vi "LS330_ReadFile.vi"(8 "error in":errorcluster, 9 "File Exists?":bool, 11 "refnum":refnum<file>) -> (0 "error out":errorcluster, 1 "Cluster":T1, 3 "refnum out":refnum<file>)   [LabVIEW 2021]
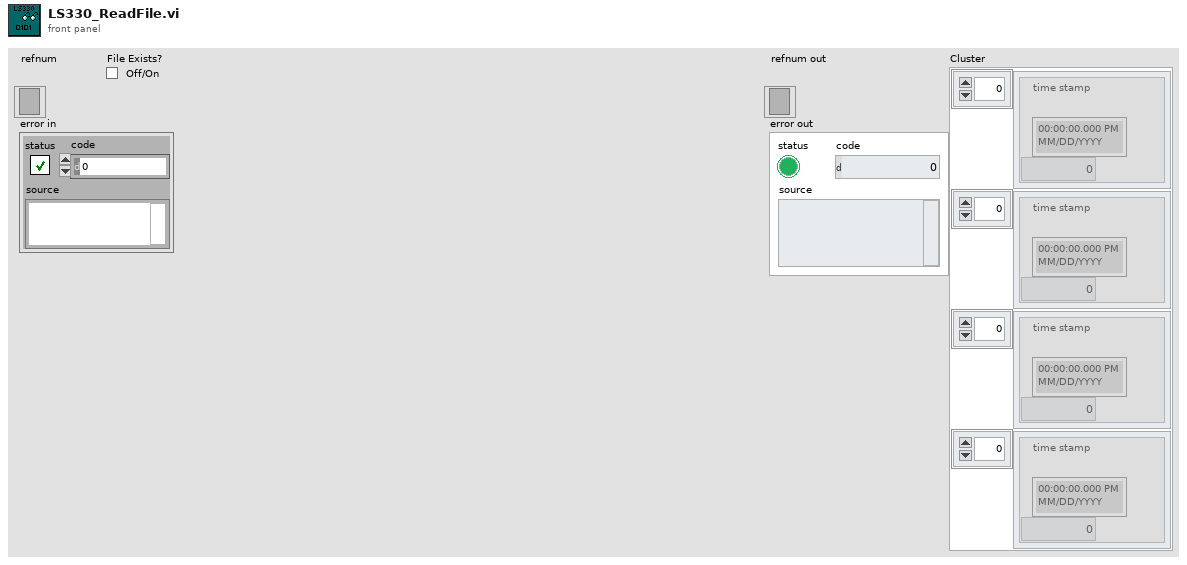
[diagram p1: front panel]
types:
  T1 = cluster{"Array":cluster{"time stamp":timestamp, "Numeric":dbl}[], "Array":cluster{"time stamp":timestamp, "Numeric":dbl}[], "Array":cluster{"time stamp":timestamp, "Numeric":dbl}[], "Array":cluster{"time stamp":timestamp, "Numeric":dbl}[]}
  T2 = cluster{cluster{"time stamp":timestamp, dbl}[], cluster{"time stamp":timestamp, dbl}[], cluster{"time stamp":timestamp, dbl}[], cluster{"time stamp":timestamp, dbl}[]}
  T3 = typedef "LVDateTimeRec.ctl" = cluster{"fractional second":dbl, "second":i32, "minute":i32, "hour":i32, "day of month":i32, "month":i32, "year":i32, "day of week":i32, "day of year":i32, "DST":i32}
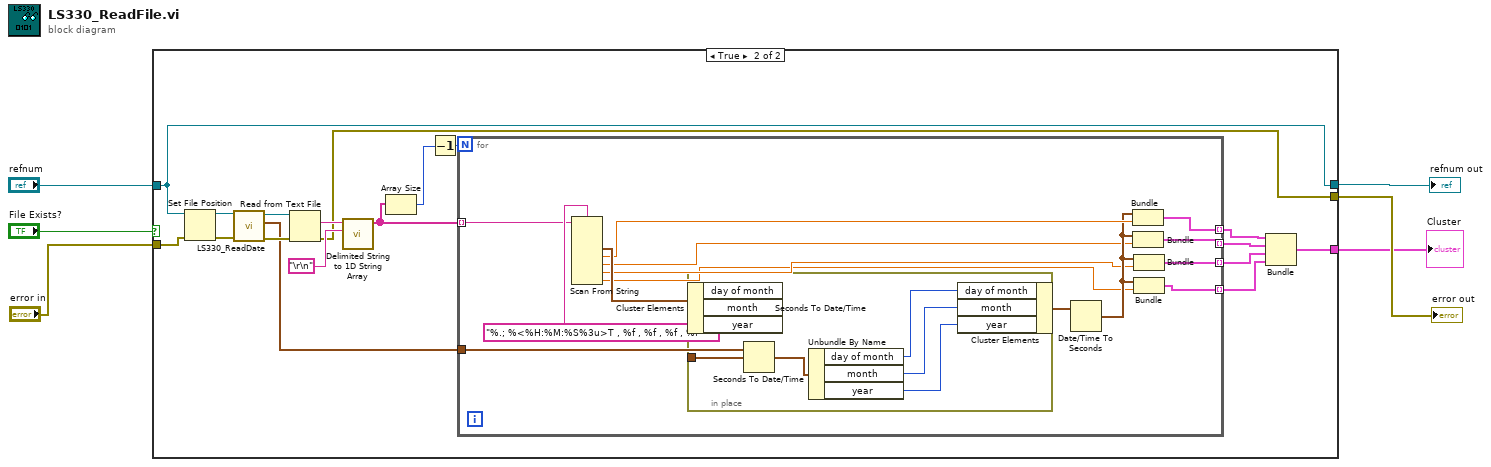
[diagram p0: block diagram]
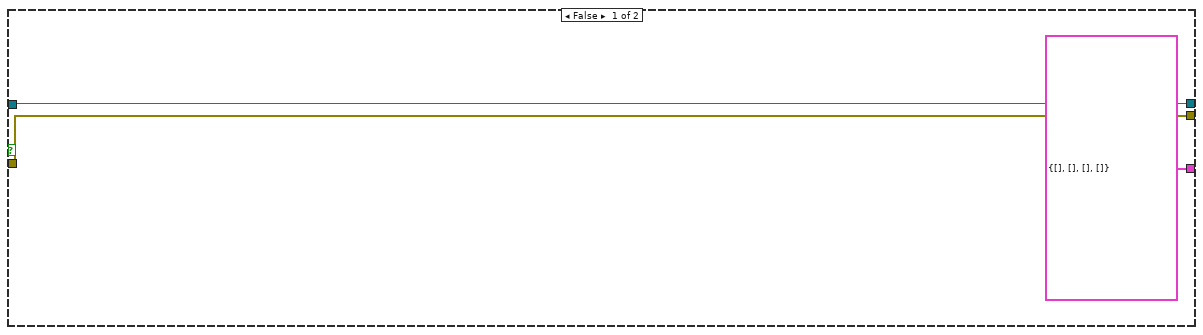
[diagram p2: hidden frame]
diagram:
  n1 = case shown="True" "File Exists?" {
    tunnel: "error in" -> [w8 w27]
    tunnel: "refnum" -> [w9 w15]
    tunnel: [w9 w15] -> w5
    tunnel: [w8 w16] -> w4
    tunnel: [T2 {[], [], [], []} w10] -> w1
    frame False {
    }
    frame True {
      n2 = Set File Position(refnum=w15, error in=w27) -> (refnum out=w26:refnum<file>, error out=w25:errorcluster)  [unwired: 2 in]
      n3 = call "LS330_ReadDate.vi"("error in"=w25, "refnum"=w26) -> ("error out"=w23:errorcluster, "Date"=w22:timestamp, "refnum 2"=w24:refnum<file>)  [unwired: 7 in]
      n4 = Read from Text File(file (use dialog)=w24, error in=w23) -> (text=w21:string, error out=w16:errorcluster)  [unwired: 2 in, 2 out]
      n5 = call <vilib>:"Delimited String to 1D String Array.vi"("delimiter"="\r\n", "delimited string"=w21) -> ("string array"=w19:string[])  [unwired: 9 in]
      n6 = Array Size(array=w19) -> (size(s)=w17:i32)
      n7 = Decrement(x=w17) -> (x-1=w18:i32)
      n8 = for {
        N: w18 -> [_]
        tunnel: w22 -> [w43]
        tunnel: w19 -> [w38] mode=indexing
        tunnel: [w36] -> w14 mode=indexing
        tunnel: [w30] -> w13 mode=indexing
        tunnel: [w29] -> w12 mode=indexing
        tunnel: [w28] -> w11 mode=indexing
        n9 = Scan From String(format string="%.; %<%H:%M:%S%3u>T , %f , %f , %f , %f", input string=w38) -> (output 1=w41:timestamp, output 2=w37:dbl, output 3=w33:dbl, output 4=w32:dbl, output 5=w31:dbl)  [unwired: 7 in, 3 out]
        n10 = Seconds To Date/Time(time stamp (now)=w41) -> (date time rec=w40:T3)  [unwired: 1 in]
        n11 = Seconds To Date/Time(time stamp (now)=w43) -> (date time rec=w39:T3)  [unwired: 1 in]
        n12 = in-place {
          in-place-border: w39 -> [w47]
          n13 = in-place-cluster #1(w40) -> ()  [unwired: 3 out]
          n14 = Unbundle By Name(w47) -> ("day of month"=w46:i32, "month"=w45:i32, "year"=w44:i32)
          n15 = in-place-cluster #1("day of month"=w46, "month"=w45, "year"=w44) -> (w35:T3)
        }
        n16 = Date/Time To Seconds(2:w35) -> (0:w34:timestamp)  [unwired: 1 in]
        n17 = Bundle("time stamp"=w34, w37) -> (w36:cluster{"time stamp":timestamp, dbl})  [unwired: 1 in]
        n18 = Bundle("time stamp"=w34, w33) -> (w30:cluster{"time stamp":timestamp, dbl})  [unwired: 1 in]
        n19 = Bundle("time stamp"=w34, w32) -> (w29:cluster{"time stamp":timestamp, dbl})  [unwired: 1 in]
        n20 = Bundle("time stamp"=w34, w31) -> (w28:cluster{"time stamp":timestamp, dbl})  [unwired: 1 in]
      }
      n21 = Bundle(w14, w13, w12, w11) -> (w10:T2)  [unwired: 1 in]
    }
  }
  "refnum out" <- w5
  "error out" <- w4
  "Cluster" <- w1
